vi "Ecg3.vi"() -> ()   [LabVIEW 2017]
uses:
  <vilib>/Math Plots/2D Math Plots/2D Feather/2D Feather XCtrl/2D Feather.xctl
  <vilib>/addons/Biomedical/Biosignal Measurements/Biosignal Preprocessing/Biosignal Rate Extractor (Waveform).vi
  <vilib>/addons/Wavelet Analysis/application.llb/WA Detrend (Waveform).vi
  <vilib>/Utility/file.llb/Read Delimited Spreadsheet (string).vi
  <vilib>/Math Plots/2D Math Plots/2D Feather/2D Feather Datatype/Public/Plot Helper (Vector).vi
  <vilib>/addons/Biomedical/NI_BMTK_Measurements.lvlib
  <vilib>/addons/_Advanced Signal Processing/NI_AdvSigProcWA.lvlib
  <vilib>/Math Plots/2D Math Plots/2D Feather/2D Feather Datatype/2D Feather Datatype.lvclass
panel:
  in  "İşle":bool
  in  "Programı sonlandır":bool
  out "Amplitude":string[](array[string])
  out "Time":string[](array[string])
  out "subarray 2":string[](array[string])
  out "subarray":string[](array[string])
  out "all rows":string[][](array[string])
  in  "Ecxel Veri okuma":path
  out "Çizgisel Grafik":refnum<class "2D Plot Datatype.lvclass">[](xcontrol) caption="2D Feather"
  in  "Path":path
  out "Kalp Atış Hızı":dbl
  out "Gürültü Engelleme":waveform(dbl)(graph)
  out "Band-Stop  Filter":dynamicdata(graph)
  out "Band-Pass Filter":dynamicdata(graph)
  out "EKG Sinyali":dynamicdata(graph)
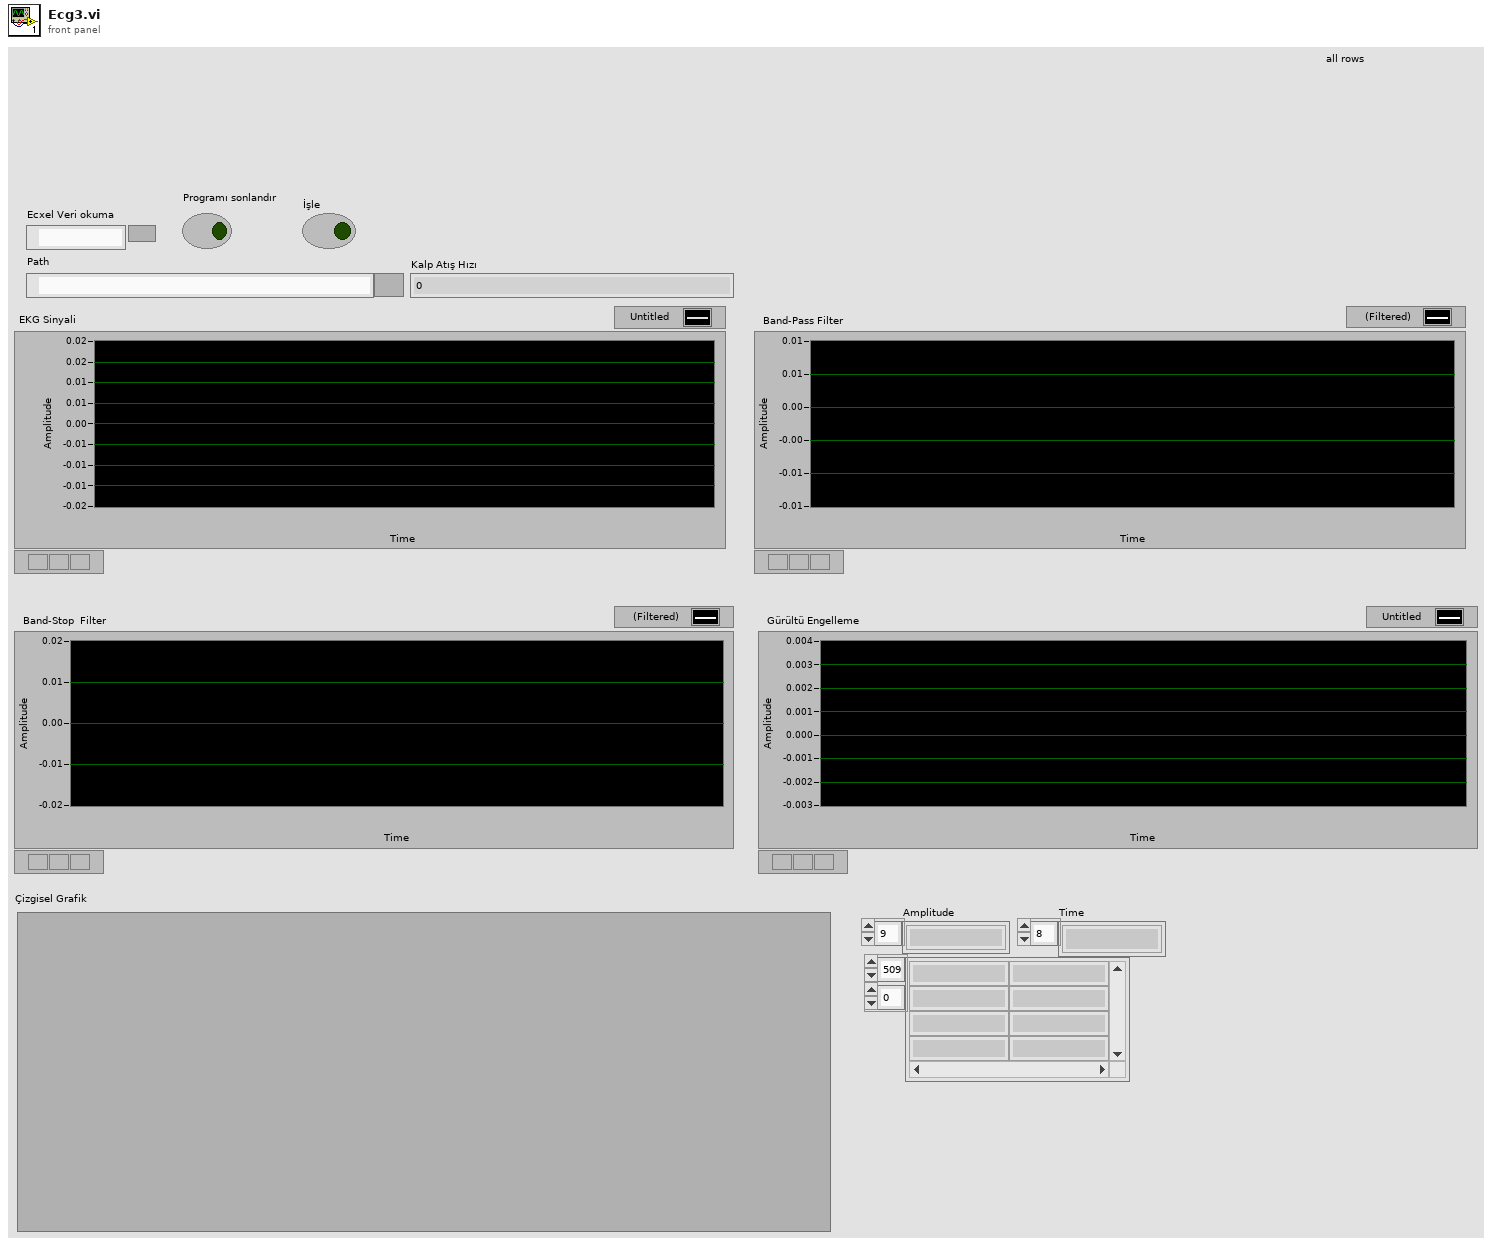
[diagram p1: front panel]
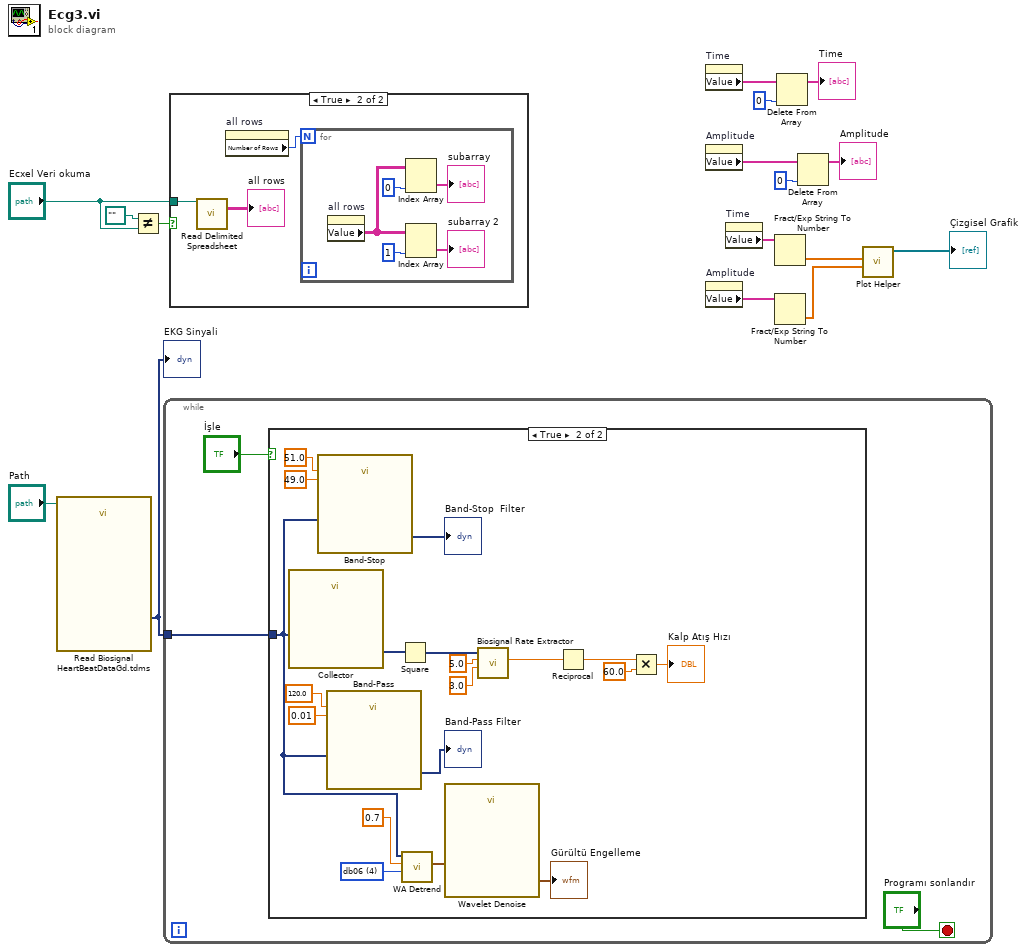
[diagram p0: block diagram]
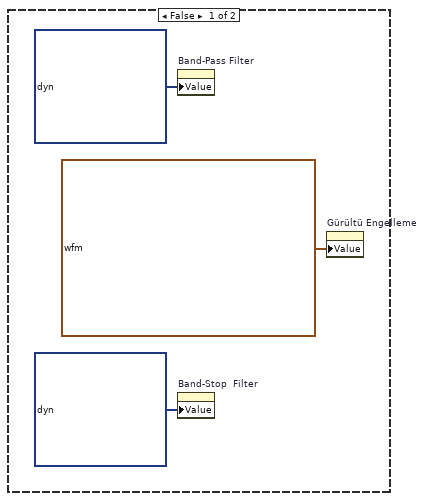
[diagram p2: hidden frame]
diagram:
  n1 = call "Read Biosignal\nHeartBeatDataGd.tdms"("file path"="Path") -> ("biosignals"=w1:dynamicdata)  [unwired: 10 in, 4 out]
  "EKG Sinyali" <- w1
  n2 = Not Equal?(x=path "" ("y"), y="Ecxel Veri okuma") -> (x != y?=w13:bool)
  n3 = while {
    tunnel: w1 -> [w17]
    stop <- "Programı sonlandır" stop-if-true
    n4 = case shown="True" "İşle" {
      tunnel: w17 -> [_ w25]
      frame False {
        n5 = property on="Band-Pass Filter" class="WFGraph (strict)"("Value"=dynamicdata [{"t0"=timestamp(0 s since 1904-01-01), "dt"=0.001, "Y"=array[1000 elements], "attributes"=variant("NI_ChannelDescription"=variant(string ""), "NI_ChannelName"=variant(string "Untitled (Filtered)"), "NI_OriginalChannelName"=variant(string "Untitled"), "NI_TSA Channel Info"=variant(cluster{"sensor sensitivity [mV/EU]":dbl, "engineering unit":u16, "custom label":string} {"sensor sensitivity [mV/EU]"=1000.0, "engineering unit"=1, "custom label"="EU"}), "NI_UnitDescription"=variant(string ""))}] ("Band-Pass Filter")) -> ()  [unwired: 2 in, 2 out]
        n6 = property on="Band-Stop  Filter" class="WFGraph (strict)"("Value"=dynamicdata [{"t0"=timestamp(0 s since 1904-01-01), "dt"=0.001, "Y"=array[1000 elements], "attributes"=variant("NI_ChannelDescription"=variant(string ""), "NI_ChannelName"=variant(string "Untitled (Filtered)"), "NI_OriginalChannelName"=variant(string "Untitled"), "NI_TSA Channel Info"=variant(cluster{"sensor sensitivity [mV/EU]":dbl, "engineering unit":u16, "custom label":string} {"sensor sensitivity [mV/EU]"=1000.0, "engineering unit"=1, "custom label"="EU"}), "NI_UnitDescription"=variant(string ""))}] ("Band-Pass Filter")) -> ()  [unwired: 2 in, 2 out]
        n7 = property on="Gürültü Engelleme" class="WFGraph (strict)"("Value"=waveform(dbl) {"t0"=timestamp(0 s since 1904-01-01), "dt"=0.001, "Y"=array[1000 elements], "attributes"=variant("NI_ChannelDescription"=variant(string ""), "NI_ChannelName"=variant(string "Untitled"), "NI_TSA Channel Info"=variant(cluster{"sensor sensitivity [mV/EU]":dbl, "engineering unit":u16, "custom label":string} {"sensor sensitivity [mV/EU]"=1000.0, "engineering unit"=1, "custom label"="EU"}), "NI_UnitDescription"=variant(string ""))} ("Gürültü Engelleme")) -> ()  [unwired: 2 in, 2 out]
      }
      frame True {
        w23 = u16 4 items=["db02"=0, "db03"=1, "db04"=2, "db05"=3, "db06"=4, "db07"=5, "db08"=6, "db09"=7, "db10"=8, "db11"=9, "db12"=10, "db13"=11, "db14"=12, "Haar"=13, "bior1_3"=14, "bior1_5"=15, "bior2_2"=16, "bior2_4"=17, "bior2_6"=18, "bior2_8"=19, "bior3_1"=20, "bior3_3"=21, "bior3_5"=22, "bior3_7"=23, "bior3_9"=24, "bior4_4 (FBI)"=25, "bior5_5"=38, "bior6_8"=39, "coif1"=26, "coif2"=27, "coif3"=28, "coif4"=29, "coif5"=30, "sym2"=31, "sym3"=32, "sym4"=33, "sym5"=34, "sym6"=35, "sym7"=36, "sym8"=37] ("wavelet")
        n8 = call "Collector"("Signals"=w25) -> ("Collected Signals"=w37:dynamicdata)  [unwired: 9 in, 1 out]
        n9 = call "Band-Stop"("Lower Cut-Off"=49.0, "Upper Cut-Off"=51.0, "Signal"=w25) -> ("Filtered Signal"=→"Band-Stop  Filter":dynamicdata)  [unwired: 7 in, 1 out]
        n10 = call "Band-Pass"("Lower Cut-Off"=0.01, "Upper Cut-Off"=120.0, "Signal"=w25) -> ("Filtered Signal"=→"Band-Pass Filter":dynamicdata)  [unwired: 7 in, 1 out]
        n11 = Square(x=w37) -> (x^2=w36:dynamicdata)
        n12 = call-poly <vilib>:"WA Detrend.vi"("wavelet"=w23, "threshold frequency"=0.7, "signal"=w25) -> ("trend signal"=w30:waveform(dbl))  [unwired: 6 in, 2 out]
        n13 = call "Wavelet Denoise"("Signal"=w30) -> ("Denoised Signal"=→"Gürültü Engelleme":waveform(dbl))  [unwired: 9 in, 1 out]
        n14 = call-poly <vilib>:"Biosignal Rate Extractor.vi"("low threshold"=3.0, "high threshold"=5.0, "biosignal"=w36) -> ("mean cycle time"=w35:dbl)  [unwired: 6 in, 2 out]
        n15 = Reciprocal(x=w35) -> (1/x=w34:dbl)
        n16 = Multiply(x=w34, y=60.0) -> (x*y=→"Kalp Atış Hızı":dbl)
      }
    }
  }
  n17 = case shown="True" w13 {
    tunnel: "Ecxel Veri okuma" -> [_ w44]
    frame False {
    }
    frame True {
      n18 = call-poly <vilib>:"Read Delimited Spreadsheet.vi"("file path (dialog if empty)"=w44) -> ("all rows"=→"all rows":string[][])  [unwired: 9 in, 5 out]
      n19 = property on="all rows" class="Arr (strict)"() -> ("Number of Rows"=w42:u32)  [unwired: 2 in, 2 out]
      n20 = for {
        N: w42 -> [_]
        n21 = property on="all rows" class="Arr (strict)"() -> ("Value"=w48:string[][])  [unwired: 2 in, 2 out]
        n22 = Index Array(array=w48, index (col)=0 ("disabled index (col)")) -> (element=→"subarray":string[])  [unwired: 1 in]
        n23 = Index Array(array=w48, index (col)=1 ("disabled index (col)")) -> (element=→"subarray 2":string[])  [unwired: 1 in]
      }
    }
  }
  n24 = property on="Time" class="Arr (strict)"() -> ("Value"=w12:string[])  [unwired: 2 in, 2 out]
  n25 = property on="Amplitude" class="Arr (strict)"() -> ("Value"=w11:string[])  [unwired: 2 in, 2 out]
  n26 = property on="Amplitude" class="Arr (strict)"() -> ("Value"=w4:string[])  [unwired: 2 in, 2 out]
  n27 = property on="Time" class="Arr (strict)"() -> ("Value"=w6:string[])  [unwired: 2 in, 2 out]
  n28 = Fract/Exp String To Number(string=w6) -> (number=w5:dbl[])  [unwired: 3 in, 1 out]
  n29 = Fract/Exp String To Number(string=w4) -> (number=w3:dbl[])  [unwired: 3 in, 1 out]
  n30 = Delete From Array(array=w12, index=0) -> (array with subset deleted=→"Time":string[])  [unwired: 1 in, 1 out]
  n31 = Delete From Array(array=w11, index=0) -> (array with subset deleted=→"Amplitude":string[])  [unwired: 1 in, 1 out]
  n32 = call-poly <vilib>:"Plot Helper.vi"("y vector"=w3, "x vector"=w5) -> ("2D Plot Class Obj Array out"=→"Çizgisel Grafik":refnum<class "2D Plot Datatype.lvclass">[])  [unwired: 2 in, 7 out]
